vi "Check_Execution_Row.vi"(0 "Execution Row":T1 {"Row Duration (mins)" format="%#.1f"; "Row No" min=0; "Trace Gas Concentration (%)" min=0.0 format="%#.2f"; "Emission Rate (l/min)" format="%#.2f"; "Tunnel Speed" format="%#.2f"; "Start X" format="%#.2f"; "Start Y" format="%#.2f"; "Start Z" format="%#.2f"; "End X" format="%#.2f"; "End Y" format="%#.2f"; "End Z" format="%#.2f"; "Averaging time (min)" min=0.0 format="%#.2f"}, 3 "Synchronization Start No":i32=1 min=1 max=100, 4 "Row Index":i32, 5 "Max Tunnel Speed":dbl format="%.2f") -> (6 "Editted Row":bool, 7 "Execution Row Out":T1 {"Row Duration (mins)" format="%#.1f"; "Row No" min=0; "Trace Gas Concentration (%)" min=0.0 format="%#.2f"; "Emission Rate (l/min)" format="%#.2f"; "Tunnel Speed" format="%#.2f"; "Start X" format="%#.2f"; "Start Y" format="%#.2f"; "Start Z" format="%#.2f"; "End X" format="%#.2f"; "End Y" format="%#.2f"; "End Z" format="%#.2f"; "Averaging time (min)" min=0.0 format="%#.2f"}, 9 "Continue?":bool, 10 "Error Comments":string)   [LabVIEW 2012]
uses:
  Traverse_cluster.ctl
  Spacing.ctl
  Controls/Multi_run_mode.ctl
  Controls/User_Specific_mode.ctl
  Controls/Tunnel_Coordinates.ctl
  ADAM Client/Sub VIs/ADAM Controls/Channel_names.ctl
  Globals/Extra_Commands_Global.vi
  Globals/Constants_global.vi
  Globals/Trav_pos_global.vi
panel:
  out "Traverse line Out":T1 {"Row Duration (mins)" format="%#.1f"; "Row No" min=0; "Trace Gas Concentration (%)" min=0.0 format="%#.2f"; "Emission Rate (l/min)" format="%#.2f"; "Tunnel Speed" format="%#.2f"; "Start X" format="%#.2f"; "Start Y" format="%#.2f"; "Start Z" format="%#.2f"; "End X" format="%#.2f"; "End Y" format="%#.2f"; "End Z" format="%#.2f"; "Averaging time (min)" min=0.0 format="%#.2f"}
  out "Fixed Axis":bool[](array[boolean])
  out "Filenames":string[](array[string])
  out "Current Sync Number":i32
  out "Checks":string[](array[string])
  in  "Edit in Excel":bool
  in  "OK":bool
  # "X           Y            Z"
  # "Start"
  # "End"
  # "X           Y            Z"
  # "Start"
  # "End"
  # "X           Y            Z"
  # "Start"
  # "End"
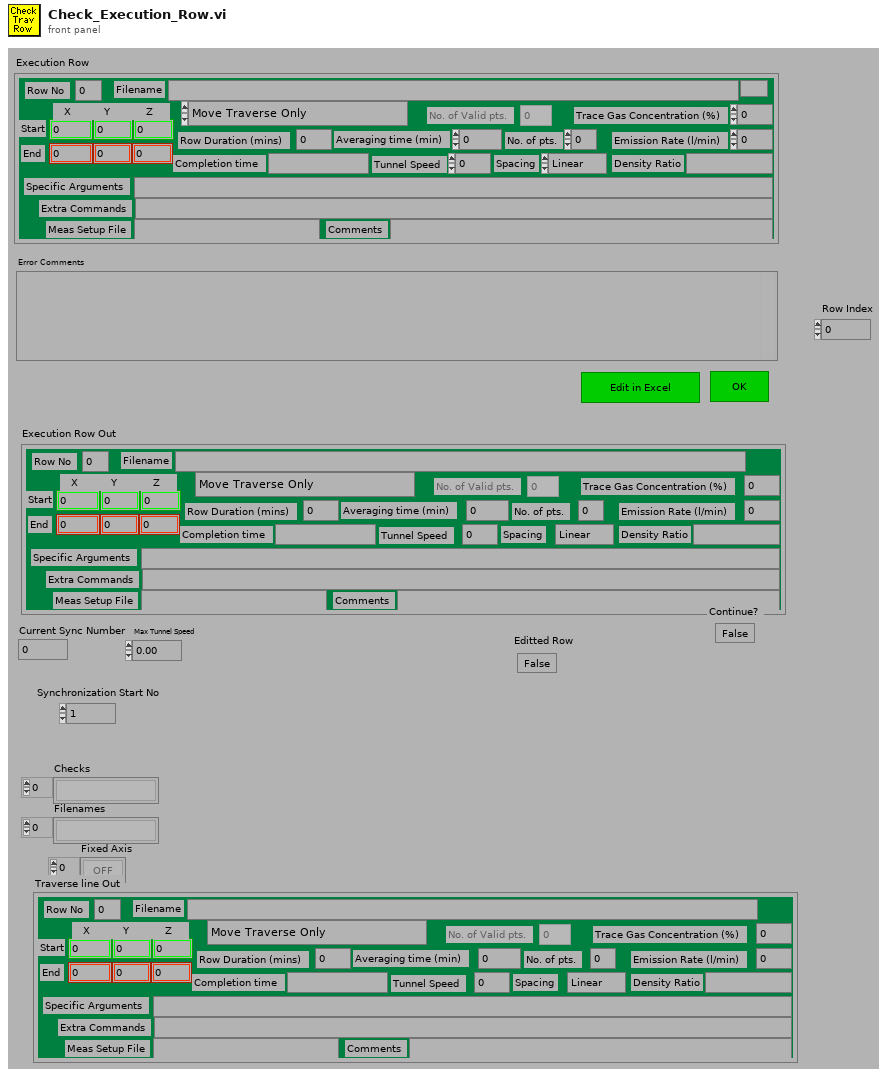
[diagram p1: front panel]
types:
  T1 = typedef "Traverse_cluster.ctl" = cluster{"Start X":dbl, "Start Y":dbl, "Start Z":dbl, "End X":dbl, "End Y":dbl, "End Z":dbl, "No. of pts.":i32, "Spacing":T2, "Filename":path, "Tunnel Speed":dbl, "Averaging time (min)":dbl, "Extra Commands":string, "Specific Arguments":string, "Emission Rate (l/min)":dbl, "Trace Gas Concentration (%)":dbl, "Density Ratio":string, "Comments":string, "Row No":i32, "Row Type Selector":T3, "Completion time":string, "Row Duration (mins)":dbl, "No. of Valid pts.":i32, "Meas Setup File":string}
  T2 = typedef "Spacing.ctl" = enum16{"Linear", "Log", "Gauss", "Specified", "N/A"}
  T3 = typedef "Multi_run_mode.ctl" = enum16{"Move Traverse Only", "Set Tunnel Speed Only", "Set Source Only", "Set Measurement Conditions", "Single Measurement", "Vertical Profile", "Lateral Profile", "Longitudinal Profile", "Explore Volume", "Multi-Axis Profile", "Auto Calibrate", "Meas Fast FID Bkgnd", "Check Beam Power", "Scanning Valve Measurement", "Run VI Named:", "Set ADAM Ch", "Wait (minutes)", "Send Message", "Synchronize With:", "Fall Back to this Row", "Turn Off Row Repeating", "Blank Row", "Traverse 3D Volume"}
  T4 = enum16{"All Channel Names", "Valid Channel Names"}
  T5 = typedef "User_Specific_mode.ctl" = enum16{"Check VI only", "Run VI"}
  T6 = typedef "Tunnel_Coordinates.ctl" = enum16{"Work in Tunnel Coordinates", "Work in Model Coordinates"}
  T7 = enum16{"Zero or one", "One", "Zero or more", "One or more"}
  T8 = typedef "Channel_names.ctl" = enum16{"Active Only", "Active + Off", "All Channels"}
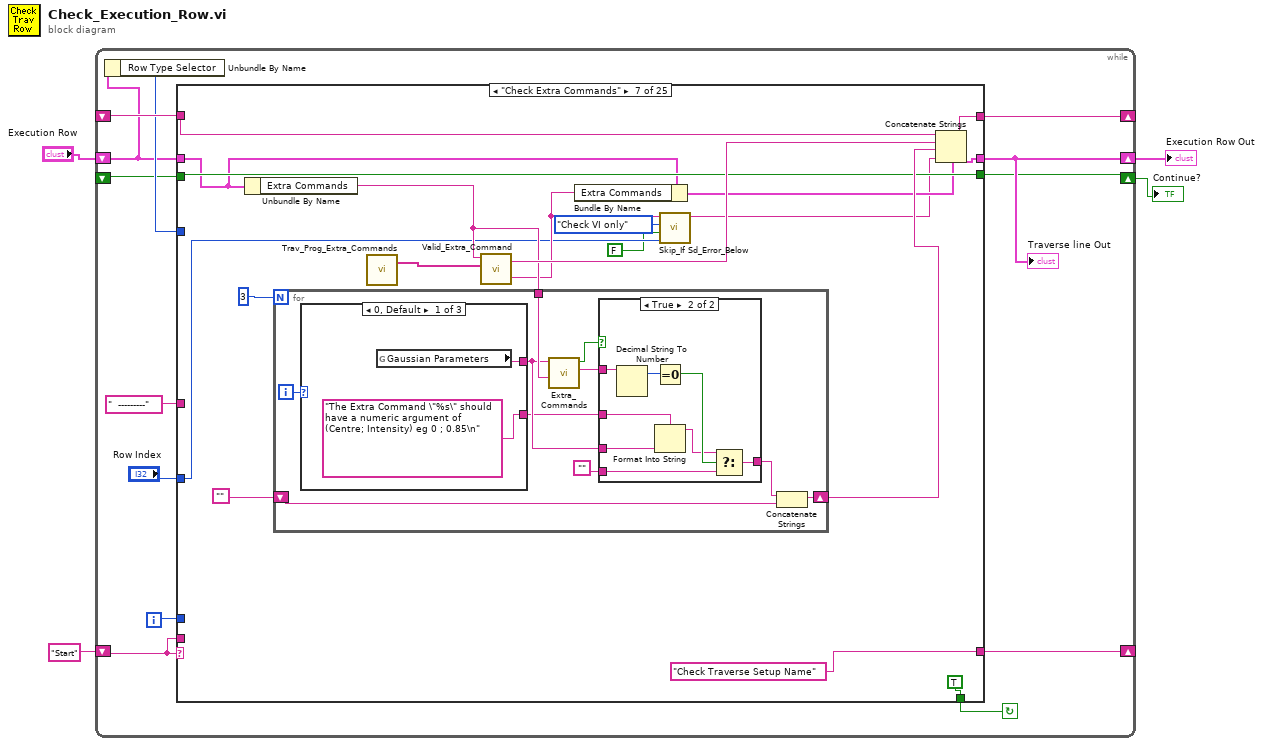
[diagram p0: block diagram]
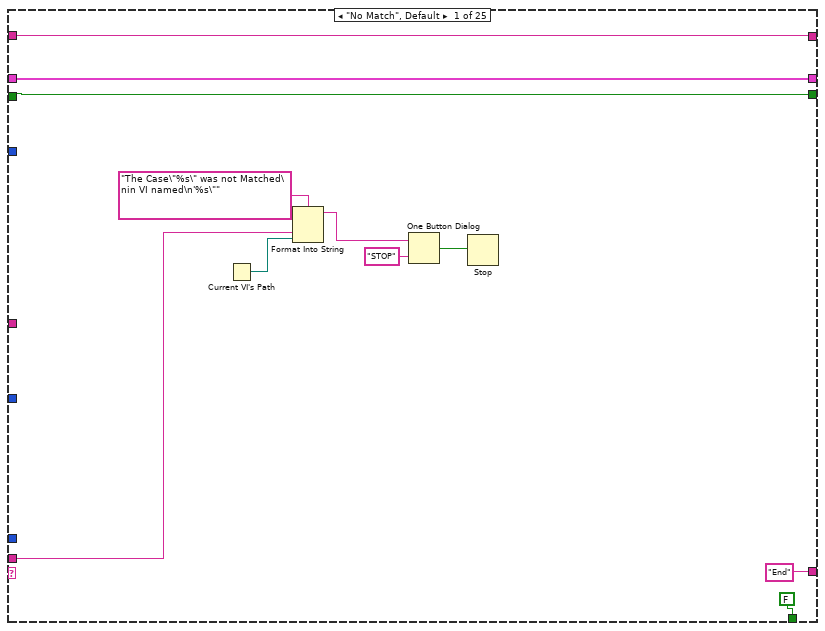
[diagram p2: hidden frame]
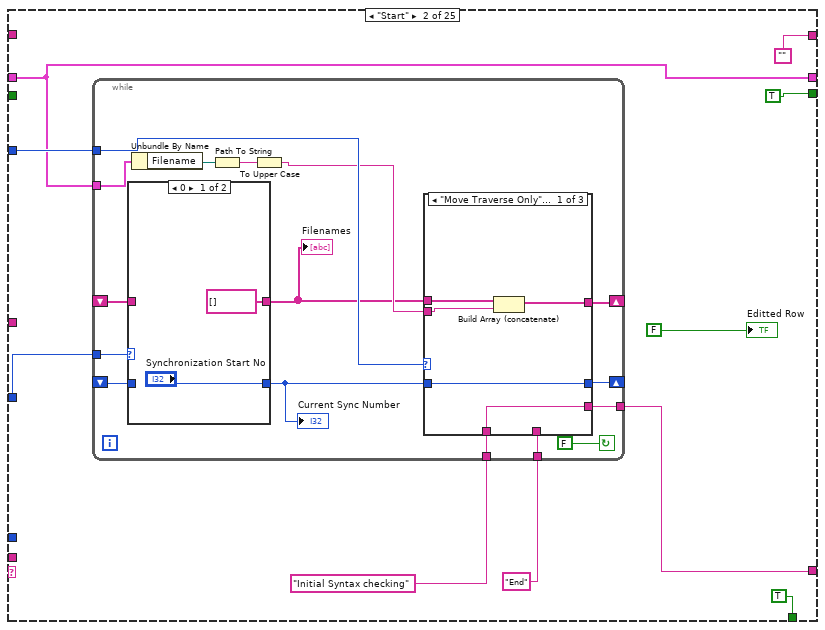
[diagram p3: hidden frame]
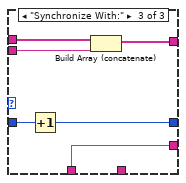
[diagram p6: hidden frame]
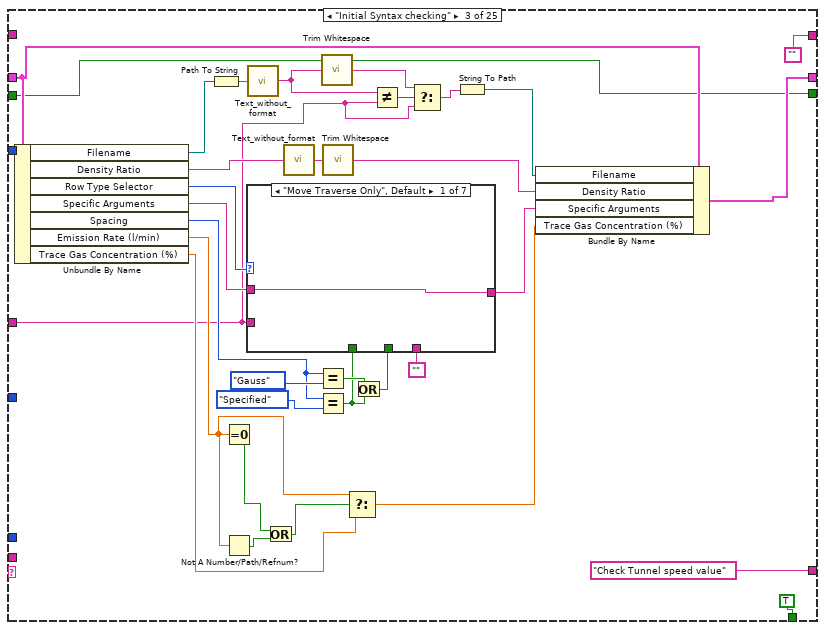
[diagram p7: hidden frame]
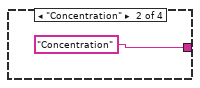
[diagram p9: hidden frame]
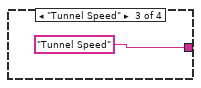
[diagram p10: hidden frame]
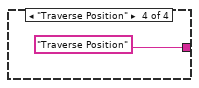
[diagram p11: hidden frame]
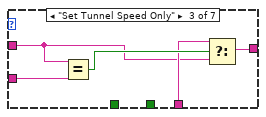
[diagram p12: hidden frame]
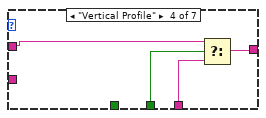
[diagram p13: hidden frame]
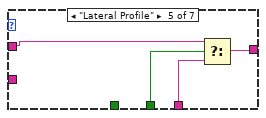
[diagram p14: hidden frame]
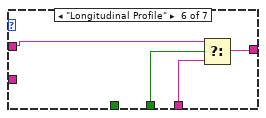
[diagram p15: hidden frame]
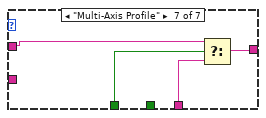
[diagram p16: hidden frame]
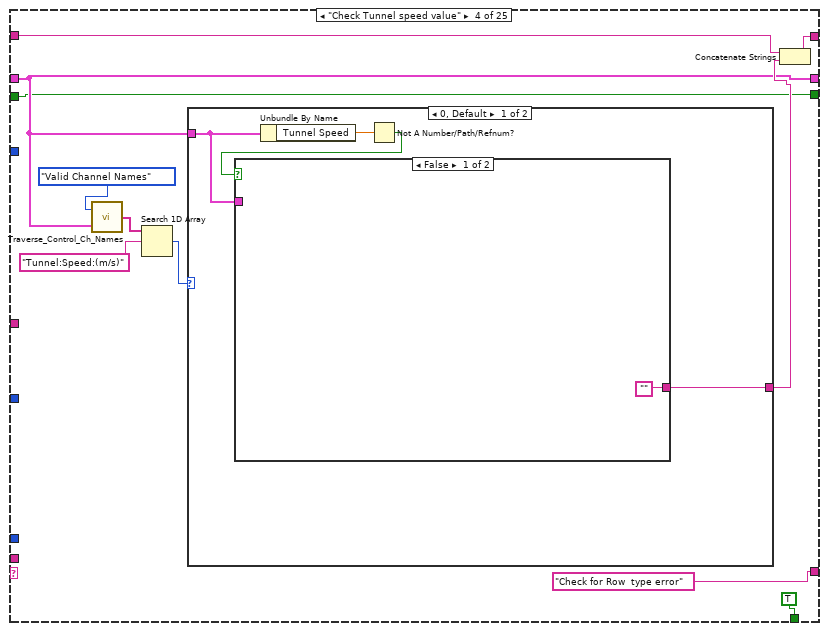
[diagram p17: hidden frame]
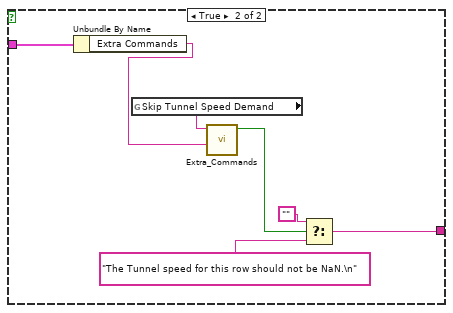
[diagram p18: hidden frame]
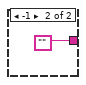
[diagram p19: hidden frame]
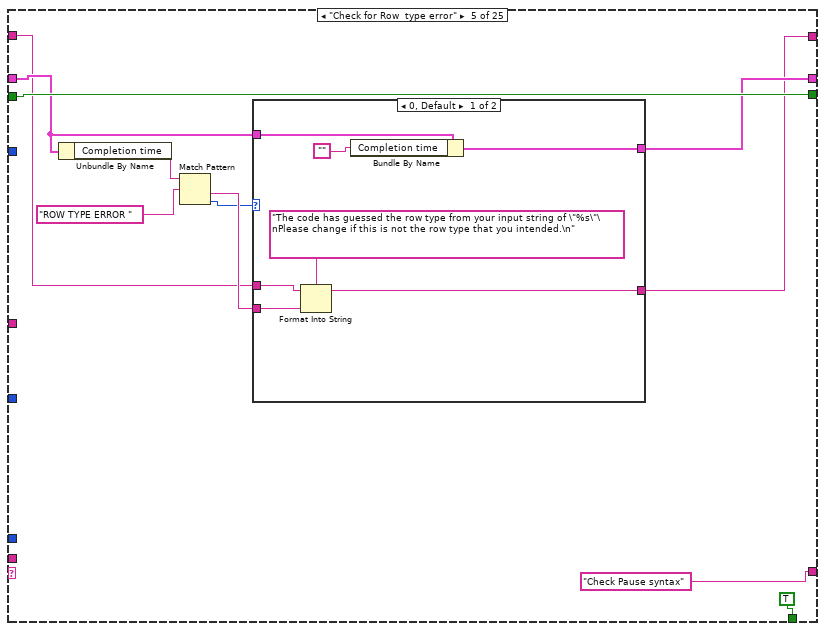
[diagram p20: hidden frame]
diagram:
  n1 = while {
    shift-left: _ -> [w16]
    shift-right: [w17] -> _
    shift-left: "Start" -> [w9]
    shift-right: [w14] -> _
    shift-right: [w8] -> w2
    shift-left: "Execution Row" -> [w5]
    shift-right: [w7] -> w1
    shift-left: _ -> [w6]
    i -> [w10]
    stop <- w15 continue-if-true
    n2 = Unbundle By Name(w5) -> ("Row Type Selector"=w12:T3)
    n3 = case shown="\"Check Extra Commands\"" w9 {
      tunnel: w5 -> [w22 w32 w100 w137 w161 w191 w205 w246 w276 w332 w365 w373 w412 w758 w858 w895 w923 w1008 w1040 w1050 w1119 _ w1158 w1165 w1175]
      tunnel: "  ---------" ("f") -> [_ _ w74 _ _ w195 _ _ _ _ _ _ _ _ _ _ _ _ _ _ _ _ _ _ _]
      tunnel: "Row Index" -> [_ w36 _ _ _ _ w202 _ _ _ _ _ w406 _ _ _ _ _ _ _ _ _ w1159 _ w1174]
      tunnel: [w21 "" "" w138 w158 w183 w213 w251 w281 w334 w369 w378 w416 w763 w868 w901 w946 w1006 w1044 w1051 w1125 w1136 w1160 w1170 w1177] -> w17
      tunnel: w12 -> [_ w35 _ _ _ _ _ _ _ _ _ w376 w415 w759 w856 _ _ _ _ w1055 _ _ _ _ _]
      tunnel: w16 -> [w21 _ _ w139 w159 w185 w214 w252 w282 w334 w368 w379 w417 w763 w869 w902 w947 w1006 w1045 w1056 w1125 w1136 w1160 w1170 w1177]
      tunnel: [FALSE TRUE TRUE TRUE TRUE TRUE TRUE TRUE TRUE TRUE TRUE TRUE TRUE TRUE TRUE TRUE TRUE TRUE TRUE w1047 TRUE TRUE TRUE TRUE FALSE] -> w15
      tunnel: ["End" w33 "Check Tunnel speed value" ("f") "Check for Row  type error" ("f") "Check Pause syntax" ("f") w188 "Check Traverse Setup Name" ("f") "Check IF command" ("f") "Check Measurement Setup?" ("f") w336 "Check Maximum tunnel speed" ("f") "Row type specific check" ("f") w413 "Check for position NaNs" ("f") w859 "Check source details" ("t") "Check source details" ("f") w1003 "check entered filename etc" ("f") w1053 "What to do next?" ("f") w1134 "Initial Syntax checking" "End" "End"] -> w14
      tunnel: w10 -> [_ _ _ _ _ _ _ _ _ _ _ _ _ _ _ _ _ _ _ _ _ _ _ _ _]
      tunnel: w9 -> [w23 _ _ _ _ _ _ _ _ _ _ _ _ _ _ _ _ _ _ _ _ _ _ _ _]
      tunnel: [w22 w32 w77 w137 w162 w178 w204 w246 w276 w332 w364 w373 w407 w757 w858 w895 w922 w1007 w1040 w1049 w1119 w1127 w1161 w1165 w1173] -> w8
      tunnel: [w18 TRUE w75 w136 w168 w179 w206 w243 w273 w338 w366 w371 w409 w755 w857 w894 w920 w1011 w1038 w1047 w1118 w1126 w1155 w1164 w1171] -> w7
      tunnel: w6 -> [w18 _ w75 w136 w168 w179 w206 w243 w273 w338 w366 w371 w409 w755 w857 w894 w920 w1011 w1038 _ w1118 _ w1155 w1164 w1171]
      frame "No Match", Default {
        n4 = Current VI's Path() -> (path=w24:path)
        n5 = Format Into String(format string="The Case\"%s\" was not Matched\nin VI named\n'%s\"" ("Format String"), w23, w24) -> (resulting string=w27:string)  [unwired: 2 in, 1 out]
        n6 = One Button Dialog(message=w27, button name ("OK")="STOP") -> (true=w25:bool)
        n7 = Stop(stop? (T)=w25) -> ()
      }
      frame "Start" {
        n8 = while {
          tunnel: "End" -> [w40]
          tunnel: "Initial Syntax checking" -> [w41]
          tunnel: [w42] -> w33
          tunnel: w32 -> [w49]
          shift-left: _ -> [w48]
          shift-right: [w47] -> _
          tunnel: w35 -> [w53]
          shift-left: _ -> [w52]
          shift-right: [w51] -> _
          tunnel: w36 -> [w54]
          stop <- FALSE continue-if-true
          n9 = case shown="0" w54 {
            tunnel: ["Synchronization Start No" w58] -> w50
            tunnel: w52 -> [_ w58]
            tunnel: w48 -> [_ w57]
            tunnel: [string[] [] w57] -> w43
            frame 0 {
            }
            frame 1, Default {
            }
          }
          "Current Sync Number" <- w50
          "Filenames" <- w43
          n10 = Unbundle By Name(w49) -> ("Filename"=w46:path)
          n11 = Path To String(path=w46) -> (string=w45:string)
          n12 = To Upper Case(1:w45) -> (0:w44:string)
          n13 = case shown="\"Move Traverse Only\", Default" w53 {
            tunnel: w50 -> [w63 w66 w72]
            tunnel: [w63 w66 w71] -> w51
            tunnel: w44 -> [w61 _ w70]
            tunnel: w43 -> [w62 w65 w69]
            tunnel: [w60 w65 w68] -> w47
            tunnel: [w59 w64 w67] -> w42
            tunnel: w41 -> [w59 _ w67]
            tunnel: w40 -> [_ w64 _]
            frame "Move Traverse Only", Default {
              n14 = Build Array (concatenate)(w62, w61) -> (w60:string[])
            }
            frame "Blank Row" {
            }
            frame "Synchronize With:" {
              n15 = Increment(x=w72) -> (x+1=w71:i32)
              n16 = Build Array (concatenate)(w69, w70) -> (w68:string[])
            }
          }
        }
        "Editted Row" <- FALSE ("Editted Row")
      }
      frame "Initial Syntax checking" {
        n17 = Unbundle By Name(w100) -> ("Filename"=w73:path, "Density Ratio"=w79:string, "Row Type Selector"=w97:T3, "Specific Arguments"=w95:string, "Spacing"=w87:T2, "Emission Rate (l/min)"=w83:dbl, "Trace Gas Concentration (%)"=w93:dbl)
        n18 = Path To String(path=w73) -> (string=w81:string)
        n19 = Equal To 0?(x=w83) -> (x = 0?=w85:bool)
        n20 = Not A Number/Path/Refnum?(number/path/refnum=w83) -> (NaN/Path/Refnum?=w84:bool)
        n21 = call "Text_without_format.vi"("Input string"=w81) -> ("Output string"=w104:string)
        n22 = Or(x=w85, y=w84) -> (x .or. y?=w82:bool)
        n23 = call "Text_without_format.vi"("Input string"=w79) -> ("Output string"=w99:string)
        n24 = Equal?(x=w87, y=Spacing."Gauss" ("Spacing")) -> (x = y?=w89:bool)
        n25 = Equal?(x=w87, y=Spacing."Specified" ("Spacing")) -> (x = y?=w86:bool)
        n26 = call <vilib>:"Trim Whitespace.vi"("string"=w104) -> ("trimmed string"=w103:string)  [unwired: 1 in]
        n27 = call <vilib>:"Trim Whitespace.vi"("string"=w99) -> ("trimmed string"=w78:string)  [unwired: 1 in]
        n28 = Select(t=w83, s=w82, f=w93) -> (s? t:f=w92:dbl)
        n29 = Or(x=w89, y=w86) -> (x .or. y?=w88:bool)
        n30 = case shown="\"Move Traverse Only\", Default" w97 {
          tunnel: [w106 w108 w113 w119 w123 w127 w131] -> w96
          tunnel: w95 -> [w106 w107 w114 w121 w125 w129 w133]
          tunnel: "" -> [_ _ w115 w120 w124 w128 w132]
          tunnel: w88 -> [_ _ _ w118 w122 w126 _]
          tunnel: w86 -> [_ _ _ _ _ _ w130]
          tunnel: w74 -> [_ _ w117 _ _ _ _]
          frame "Move Traverse Only", Default {
          }
          frame "Auto Calibrate" {
            n31 = case shown="\"No Match\", Default" w107 {
              tunnel: [w109 "Concentration" "Tunnel Speed" "Traverse Position"] -> w108
              tunnel: w107 -> [w109 _ _ _]
              frame "No Match", Default {
              }
              frame "Concentration" {
              }
              frame "Tunnel Speed" {
              }
              frame "Traverse Position" {
              }
            }
          }
          frame "Set Tunnel Speed Only" {
            n32 = Equal?(x=w114, y=w117) -> (x = y?=w116:bool)
            n33 = Select(t=w115, s=w116, f=w114) -> (s? t:f=w113:string)
          }
          frame "Vertical Profile" {
            n34 = Select(t=w121, s=w118, f=w120) -> (s? t:f=w119:string)
          }
          frame "Lateral Profile" {
            n35 = Select(t=w125, s=w122, f=w124) -> (s? t:f=w123:string)
          }
          frame "Longitudinal Profile" {
            n36 = Select(t=w129, s=w126, f=w128) -> (s? t:f=w127:string)
          }
          frame "Multi-Axis Profile" {
            n37 = Select(t=w133, s=w130, f=w132) -> (s? t:f=w131:string)
          }
        }
        n38 = Not Equal?(x=w104, y=w74) -> (x != y?=w105:bool)
        n39 = Select(t=w103, s=w105, f=w74) -> (s? t:f=w102:string)
        n40 = String To Path(string=w102) -> (path=w80:path)
        n41 = Bundle By Name(cluster=w100, "Filename"=w80, "Density Ratio"=w78, "Specific Arguments"=w96, "Trace Gas Concentration (%)"=w92) -> (w77:T1)
      }
      frame "Check Tunnel speed value" {
        n42 = call "Traverse_Control_Ch_Names.vi"("Traverse line"=w137, "Mode"=T4."Valid Channel Names") -> ("Channel names"=w143:string[])
        n43 = Search 1D Array(1D array=w143, element="Tunnel:Speed:(m/s)" ("Label for value")) -> (index of element=w141:i32)  [unwired: 1 out]
        n44 = case shown="0, Default" w141 {
          tunnel: w137 -> [w146 _]
          tunnel: [w145 ""] -> w140
          frame 0, Default {
            n45 = Unbundle By Name(w146) -> ("Tunnel Speed"=w148:dbl)
            n46 = Not A Number/Path/Refnum?(number/path/refnum=w148) -> (NaN/Path/Refnum?=w147:bool)
            n47 = case shown="False" w147 {
              tunnel: w146 -> [_ w156]
              tunnel: ["" w150] -> w145
              frame False {
              }
              frame True {
                n48 = Unbundle By Name(w156) -> ("Extra Commands"=w154:string)
                n49 = global read "Extra_Commands_Global.vi" "Skip Tunnel Speed Demand"() -> (w155:string)
                n50 = call "Extra_Commands.vi"("String to Search"=w154, "Command"=w155) -> ("Command Found"=w153:bool)  [unwired: 1 in, 4 out]
                n51 = Select(t="", s=w153, f="The Tunnel speed for this row should not be NaN.\n") -> (s? t:f=w150:string)
              }
            }
          }
          frame -1 {
          }
        }
        n52 = Concatenate Strings(w139, w140) -> (w138:string)
      }
      frame "Check for Row  type error" {
        n53 = Unbundle By Name(w161) -> ("Completion time"=w164:string)
        n54 = Match Pattern(string=w164, regular expression="ROW TYPE ERROR " ("format string")) -> (after substring=w163:string, offset past match=w160:i32)  [unwired: 3 out]
        n55 = case shown="0, Default" w160 {
          tunnel: w163 -> [w175 _]
          tunnel: [w173 w177] -> w162
          tunnel: w161 -> [w172 w177]
          tunnel: [w170 w176] -> w158
          tunnel: w159 -> [w169 w176]
          frame 0, Default {
            n56 = Format Into String(format string="The code has guessed the row type from your input string of \"%s\"\nPlease change if this is not the row type that you intended.\n", initial string=w169, w175) -> (resulting string=w170:string)  [unwired: 1 in, 1 out]
            n57 = Bundle By Name(cluster=w172, "Completion time"="") -> (w173:T1)
          }
          frame -1 {
          }
        }
      }
      frame "Check Pause syntax" {
        n58 = Unbundle By Name(w191) -> ("Extra Commands"=w196:string)
        n59 = Not Equal?(x=w196, y=w195) -> (x != y?=w197:bool)
        n60 = Select(t=w196, s=w197, f="") -> (s? t:f=w193:string)
        n61 = call <vilib>:"Trim Whitespace.vi"("string"=w193) -> ("trimmed string"=w187:string)  [unwired: 1 in]
        n62 = Equal?(x=w187, y="") -> (x = y?=w189:bool)
        n63 = call "Pause_for_server_ch_val.vi"("Extra command string"=w187, "Simulate/Run"=User_Specific_mode."Check VI only") -> ("Extra command string Out"=w186:string, "Error Comments"=w184:string)
        n64 = Bundle By Name(cluster=w191, "Extra Commands"=w186) -> (w178:T1)
        n65 = Concatenate Strings(w185, w184) -> (w183:string)
        n66 = Select(t="Check Measurement Setup?", s=w189, f="Check Extra Commands") -> (s? t:f=w188:string)
      }
      frame "Check Extra Commands" {
        n67 = Unbundle By Name(w205) -> ("Extra Commands"=w207:string)
        n68 = for {
          N: 3 -> [_]
          tunnel: w207 -> [w222]
          shift-right: [w218] -> w210
          shift-left: "" -> [w219]
          i -> [w224]
          n69 = case shown="0, Default" w224 {
            tunnel: [w227 w229 w231] -> w221
            tunnel: ["The Extra Command \"%s\" should have a numeric argument of (Centre; Intensity) eg 0 ; 0.85\n" ("Format String") "The Extra Command \"%s\" should have a numeric argument.\n" ("Format String") "The Extra Command \"%s\" should have a numeric argument.\n" ("Format String")] -> w216
            frame 0, Default {
              n70 = global read "Extra_Commands_Global.vi" "Gaussian Parameters"() -> (w227:string)
            }
            frame 1 {
              n71 = global read "Extra_Commands_Global.vi" "Establish Exp Conditions (s)"() -> (w229:string)
            }
            frame 2 {
              n72 = global read "Extra_Commands_Global.vi" "Minutes Before Repeating Row"() -> (w231:string)
            }
          }
          n73 = call "Extra_Commands.vi"("String to Search"=w222, "Command"=w221) -> ("String Value"=w223:string, "Command Found"=w225:bool)  [unwired: 1 in, 3 out]
          n74 = case shown="True" w225 {
            tunnel: w223 -> [_ w240]
            tunnel: w221 -> [_ w238]
            tunnel: [w232 w235] -> w220
            tunnel: "" -> [w232 w234]
            tunnel: w216 -> [_ w233]
            frame False {
            }
            frame True {
              n75 = Decimal String To Number(string=w240) -> (offset past number=w239:i32)  [unwired: 3 out]
              n76 = Equal To 0?(x=w239) -> (x = 0?=w237:bool)
              n77 = Format Into String(format string=w233, w238) -> (resulting string=w236:string)  [unwired: 2 in, 1 out]
              n78 = Select(t=w236, s=w237, f=w234) -> (s? t:f=w235:string)
            }
          }
          n79 = Concatenate Strings(w220, w219) -> (w218:string)
        }
        n80 = call "Trav_Prog_Extra_Commands.vi"() -> ("Extra Commands Array"=w208:string[])  [unwired: 2 out]
        n81 = call "Valid_Extra_Command.vi"("Extra Commands string"=w207, "Valid Commands Array"=w208) -> ("Output String"=w212:string, "Extra Commands string Out"=w203:string)  [unwired: 3 out]
        n82 = Bundle By Name(cluster=w205, "Extra Commands"=w203) -> (w204:T1)
        n83 = call "Skip_If Sd_Error_Below.vi"("String to Search"=w203, "Simulate/Run"=User_Specific_mode."Check VI only", "Measurement setup Applied?"=FALSE, "Row Number"=w202) -> ("Error String"=w199:string)  [unwired: 1 in, 4 out]
        n84 = Concatenate Strings(w214, w212, w210, w199) -> (w213:string)
      }
      frame "Check Traverse Setup Name" {
        n85 = Unbundle By Name(w246) -> ("Extra Commands"=w242:string)
        n86 = global read "Extra_Commands_Global.vi" "!Traverse Setup"() -> (w249:string)
        n87 = call "Extra_Commands.vi"("String to Search"=w242, "Command"=w249) -> ("String Value"=w247:string, "Command Found"=w248:bool)  [unwired: 1 in, 3 out]
        n88 = case shown="True" w248 {
          tunnel: w247 -> [_ w259]
          tunnel: [w253 w256] -> w244
          tunnel: "" -> [w253 w255]
          frame False {
          }
          frame True {
            n89 = global read "Constants_global.vi" "Traverse folder"() -> (w254:path)
            n90 = List Folder(path=w254) -> (folder names=w257:string[])  [unwired: 1 in, 5 out]
            n91 = Search 1D Array(1D array=w257, element=w259) -> (index of element=w260:i32)  [unwired: 1 out]
            n92 = Greater Or Equal To 0?(x=w260) -> (x >= 0?=w258:bool)
            n93 = case shown="False" w258 {
              tunnel: w259 -> [w265 _]
              tunnel: w257 -> [w262 _]
              tunnel: [w261 w270] -> w256
              tunnel: w255 -> [_ w270]
              frame False {
                n94 = Format Into String(format string="%s is not a valid Travese setup. Valid option are:", w265) -> (resulting string=w263:string)  [unwired: 2 in, 1 out]
                n95 = for {
                  shift-right: [w267] -> w261
                  shift-left: w263 -> [w268]
                  tunnel: w262 -> [w269] mode=indexing
                  w266 = "  " ("Substring")
                  n96 = Concatenate Strings(w268, w266, w269, w266) -> (w267:string)
                }
              }
              frame True {
              }
            }
          }
        }
        n97 = Concatenate Strings(w252, w244) -> (w251:string)
      }
      frame "Check IF command" {
        n98 = Unbundle By Name(w276) -> ("Extra Commands"=w272:string)
        n99 = global read "Extra_Commands_Global.vi" "If Command"() -> (w279:string)
        n100 = call "Extra_Commands.vi"("String to Search"=w272, "Command"=w279) -> ("String Value"=w277:string, "Command Found"=w278:bool)  [unwired: 1 in, 3 out]
        n101 = case shown="True" w278 {
          tunnel: w277 -> [_ w288]
          tunnel: [w283 w287] -> w274
          tunnel: "" -> [w283 w285]
          frame False {
          }
          frame True {
            n102 = call "Get_array_values_fr_String.vi"("String Value"=w288) -> ("Numeric Array"=w284:dbl[], "String array"=w286:string[])
            n103 = Index Array(array=w286, index=0 ("Index")) -> (element=w289:string)
            n104 = case shown="\"Global Value Between\"" w289 {
              tunnel: w288 -> [w294 _ _ _]
              tunnel: [w293 w319 w320 "The !If  command has not been recognised.\nExtra command Example:\n!IF = Time Between;10:45;and;14:00;Execute Row (or) Skip Row\n\n!IF = ADAM Channel Between;Channel Name; 0.5;1.0\n\n!IF = Global Value Between; 0.5;1.0" ("Error Comments")] -> w287
              tunnel: w286 -> [_ w310 w328 _]
              tunnel: w285 -> [_ w303 w321 _]
              tunnel: w284 -> [_ _ _ _]
              frame "Time Between" {
                n105 = Get Date/Time In Seconds() -> (seconds since 1Jan1904=w291:timestamp)
                n106 = To Double Precision Float(number=w291) -> (double precision float=w292:dbl)
                n107 = call "If_Time_arguments.vi"("seconds since 1Jan1904"=w292, "String Value"=w294) -> ("Error Comments"=w293:string)  [unwired: 2 out]
              }
              frame "ADAM Channel Between" {
                n108 = Index Array(array=w310, index=1 ("Index")) -> (element=w313:string)
                n109 = Index Array(array=w310, index=2 ("Index")) -> (element=w309:string)
                n110 = Index Array(array=w310, index=3 ("Index")) -> (element=w308:string)
                n111 = Build Array(w313) -> (w315:string[])
                n112 = Decimal Digit?(1:w309) -> (0:w306:bool)
                n113 = Decimal Digit?(1:w308) -> (0:w307:bool)
                n114 = call "Get_Current_Scan_client.vi"("ADAM Ch Names"=w315) -> ("Numerical Values"=w317:dbl[])  [unwired: 3 out]
                n115 = And(x=w306, y=w307) -> (x .and. y?=w305:bool)
                n116 = Index Array(array=w317, index=0 ("Index")) -> (element=w318:dbl)
                n117 = Select(t=w303, s=w305, f="you must give two limits\n") -> (s? t:f=w299:string)
                n118 = Not A Number/Path/Refnum?(number/path/refnum=w318) -> (NaN/Path/Refnum?=w302:bool)
                n119 = Select(t="Invalid ADAM Channel Name\n", s=w302, f=w303) -> (s? t:f=w300:string)
                n120 = Concatenate Strings(w300, w299) -> (w297:string)
                n121 = Concatenate Strings(w297, "Extra command Example:\n!IF = ADAM Channel Between;Channel Name; 0.5;1.0") -> (w296:string)
                n122 = Empty String/Path?(string/path=w297) -> (empty?=w298:bool)
                n123 = Select(t=w303, s=w298, f=w296) -> (s? t:f=w319:string)
              }
              frame "Global Value Between" {
                n124 = Index Array(array=w328, index=1 ("Index")) -> (element=w327:string)
                n125 = Index Array(array=w328, index=2 ("Index")) -> (element=w326:string)
                n126 = Decimal Digit?(1:w327) -> (0:w324:bool)
                n127 = Decimal Digit?(1:w326) -> (0:w325:bool)
                n128 = And(x=w324, y=w325) -> (x .and. y?=w323:bool)
                n129 = Select(t=w321, s=w323, f="The Extra command IF statement must have two numerical values for the limits\n\nExtra command Example:\n!IF = Global Value Between; 0.5;1.0") -> (s? t:f=w320:string)
              }
              frame "No Match", Default {
              }
            }
          }
        }
        n130 = Concatenate Strings(w282, w274) -> (w281:string)
      }
      frame "Check Measurement Setup?" {
        n131 = Unbundle By Name(w332) -> ("Row Type Selector"=w337:T3, "Specific Arguments"=w335:string)
        n132 = case shown="\"Traverse 3D Volume\"" w337 {
          tunnel: ["Check Measurement Setup" ("t") "Check Measurement Setup" ("t") "Check Measurement Setup" ("t") "Check Measurement Setup" ("t") "Check Measurement Setup" ("t") "Check Measurement Setup" ("t") "Check Measurement Setup" ("t") "Check Measurement Setup" ("t") "Check Measurement Setup" ("t") "Check Measurement Setup" ("t") "Check Measurement Setup" ("t") w351 w360] -> w336
          tunnel: w335 -> [_ _ _ _ _ _ _ _ _ _ _ w358 _]
          tunnel: "Check Maximum tunnel speed" ("f") -> [_ _ _ _ _ _ _ _ _ _ _ w352 w360]
          tunnel: w332 -> [_ _ _ _ _ _ _ _ _ _ _ w355 _]
          frame "Lateral Profile" {
          }
          frame "Traverse 3D Volume" {
          }
          frame "Longitudinal Profile" {
          }
          frame "Explore Volume" {
          }
          frame "Multi-Axis Profile" {
          }
          frame "Vertical Profile" {
          }
          frame "Single Measurement" {
          }
          frame "Scanning Valve Measurement" {
          }
          frame "Auto Calibrate" {
          }
          frame "Meas Fast FID Bkgnd" {
          }
          frame "Check Beam Power" {
          }
          frame "Run VI Named:" {
            n133 = Match Pattern(string=w358, regular expression=";") -> (before substring=w357:string)  [unwired: 4 out]
            n134 = call <vilib>:"Trim Whitespace.vi"("string"=w357) -> ("trimmed string"=w356:string)  [unwired: 1 in]
            n135 = call "Run_VI_Named_specific.vi"("Run VI Named String"=w356, "Multi Run Row"=w355) -> ("Check Meas Setup?"=w354:bool)  [unwired: 9 out]
            n136 = Select(t="Check Measurement Setup", s=w354, f=w352) -> (s? t:f=w351:string)
          }
          frame "Set Tunnel Speed Only", Default {
          }
        }
      }
      frame "Check Measurement Setup" {
        n137 = Unbundle By Name(w365) -> ("Meas Setup File"=w363:string)
        n138 = call "Check_Measurement_Setups.vi"("Measurement Setup String"=w363) -> ("Measurement Setup String Out"=w362:string, "Error Comments"=w361:string)
        n139 = Bundle By Name(cluster=w365, "Meas Setup File"=w362) -> (w364:T1)
        n140 = Concatenate Strings(w368, w361) -> (w369:string)
      }
      frame "Check Maximum tunnel speed" {
        n141 = case shown="\"Set Tunnel Speed Only\", Default" w376 {
          tunnel: w373 -> [w398 _]
          tunnel: [w389 FALSE] -> w375
          tunnel: [w388 0.0] -> w374
          frame "Auto Calibrate" {
            n142 = Unbundle By Name(w398) -> ("Specific Arguments"=w397:string)
            n143 = call "Get_array_values_fr_String.vi"("String Value"=w397) -> ("Numeric Array"=w391:dbl[], "String array"=w396:string[])
            n144 = Index Array(array=w396, index=0 ("Index")) -> (element=w394:string)
            n145 = Equal?(x=w394, y="Tunnel Speed" ("Output Array")) -> (x = y?=w389:bool)
            n146 = Array Subset(array=w391, index=1 ("Array Index")) -> (w390:dbl[])  [unwired: 1 in]
            n147 = Array Max & Min(array=w390) -> (max value=w388:dbl)  [unwired: 3 out]
          }
          frame "Set Tunnel Speed Only", Default {
          }
        }
        n148 = case shown="False" w375 {
          tunnel: [w386 w387] -> w383
          tunnel: w373 -> [w385 _]
          tunnel: w374 -> [_ w387]
          frame False {
            n149 = Unbundle By Name(w385) -> ("Tunnel Speed"=w386:dbl)
          }
          frame True {
          }
        }
        n150 = Greater?(x=w383, y="Max Tunnel Speed") -> (0:w381:bool)
        n151 = Not A Number/Path/Refnum?(number/path/refnum=w383) -> (NaN/Path/Refnum?=w382:bool)
        n152 = Compound Arithmetic op=AND(invert w382, w381) -> (w380:bool)
        n153 = case shown="False" w380 {
          tunnel: w379 -> [w401 w403]
          tunnel: [w401 w402] -> w378
          tunnel: "Max Tunnel Speed" -> [_ w405]
          frame False {
          }
          frame True {
            n154 = Format Into String(format string="The maximum allowable tunnel speed is %.2f m/s.\n" ("Format String"), initial string=w403, w405) -> (resulting string=w402:string)  [unwired: 1 in, 1 out]
          }
        }
      }
      frame "Row type specific check" {
        n155 = case shown="\"Check Beam Power\"" w415 {
          tunnel: w412 -> [w426 w435 w439 w443 w448 w453 w460 w467 w478 w486 w500 w504 w581 w588 w609 w637 w686 w714 w719 w723 w735 w739 w745]
          tunnel: [string[] [] string[] [] string[] [] string[] [] w449 w456 w463 w470 w483 w491 w501 w526 w583 string[] [] w626 string[] [] w681 string[] [] string[] [] string[] [] string[] [] string[] [] string[] []] -> w414
          tunnel: [w420 "" "" "" "" "" "" "" w479 w488 "" w540 w577 w587 w621 w629 w697 w716 "" w725 "" "" w747] -> w418
          tunnel: [w429 w436 w440 w444 w447 w454 w461 w468 w477 w487 w499 w525 w571 w586 w620 w640 w682 "check entered filename etc" "check entered filename etc" "check entered filename etc" "check entered filename etc" "check entered filename etc" "check entered filename etc"] -> w413
          tunnel: "Check source details" -> [_ w436 w440 _ _ _ _ _ _ _ w499 _ w571 w586 w620 w639 w683 _ _ _ _ _ _]
          tunnel: "Sort out start and end positions" -> [_ _ _ _ _ w454 w461 w468 _ w487 _ w523 _ _ _ _ _ _ _ _ _ _ _]
          tunnel: "Check for Start NaNs" -> [w429 _ _ w444 w447 _ _ _ w477 _ _ w524 _ _ _ _ _ _ _ _ _ _ _]
          tunnel: [w425 w435 w439 w443 w448 w453 w460 w467 w478 w486 w500 w505 w581 w596 w609 w636 w686 w714 w719 w723 w735 w739 w743] -> w407
          tunnel: w406 -> [_ _ _ _ _ _ _ _ _ _ _ _ _ _ _ w642 _ _ _ _ _ _ _]
          frame "Move Traverse Only" {
            n156 = Unbundle By Name(w426) -> ("Specific Arguments"=w427:string)
            n157 = call <vilib>:"Trim Whitespace.vi"("string"=w427) -> ("trimmed string"=w421:string)  [unwired: 1 in]
            n158 = Equal?(x=w421, y="No Backlash") -> (x = y?=w424:bool)
            n159 = Empty String/Path?(string/path=w421) -> (empty?=w423:bool)
            n160 = Or(x=w423, y=w424) -> (x .or. y?=w422:bool)
            n161 = case shown="True" w422 {
              tunnel: w421 -> [w432 _]
              tunnel: [w431 ""] -> w420
              frame False {
                n162 = Format Into String(format string="\"%s\" is an Incorrect Specific Argument. It should either be left blank or say \"No Backlash\"\n", w432) -> (resulting string=w431:string)  [unwired: 2 in, 1 out]
              }
              frame True {
              }
            }
            n163 = Bundle By Name(cluster=w426, "Specific Arguments"=w421) -> (w425:T1)
          }
          frame "Set Tunnel Speed Only" {
          }
          frame "Set Source Only" {
          }
          frame "Set Measurement Conditions" {
          }
          frame "Single Measurement" {
            n164 = Build Array("Averaging:Time:(mins)" ("Label for value"), "Filename:HD:Users" ("Label for value")) -> (w449:string[])
          }
          frame "Vertical Profile" {
            n165 = Build Array("Number:Of:Points" ("Label for value"), "Averaging:Time:(mins)" ("Label for value"), "Filename:HD:Users" ("Label for value")) -> (w456:string[])
          }
          frame "Lateral Profile" {
            n166 = Build Array("Number:Of:Points" ("Label for value"), "Averaging:Time:(mins)" ("Label for value"), "Filename:HD:Users" ("Label for value")) -> (w463:string[])
          }
          frame "Longitudinal Profile" {
            n167 = Build Array("Number:Of:Points" ("Label for value"), "Averaging:Time:(mins)" ("Label for value"), "Filename:HD:Users" ("Label for value")) -> (w470:string[])
          }
          frame "Explore Volume" {
            n168 = Unbundle By Name(w478) -> ("Specific Arguments"=w476:string)
            n169 = Build Array("Averaging:Time:(mins)" ("Label for value"), "Filename:HD:Users" ("Label for value")) -> (w483:string[])
            n170 = Fract/Exp String To Number(string=w476) -> (number=w475:dbl)  [unwired: 4 out]
            n171 = Greater Than 0?(x=w475) -> (x > 0?=w474:bool)
            n172 = Format Into String(format string="\"%s\" is an Incorrect Specific Argument. Please enter the radius of the volume in mm.\n", w476) -> (resulting string=w480:string)  [unwired: 2 in, 1 out]
            n173 = Select(t="", s=w474, f=w480) -> (s? t:f=w479:string)
          }
          frame "Multi-Axis Profile" {
            n174 = Unbundle By Name(w486) -> ("Spacing"=w489:T2)
            n175 = case shown="\"Gauss\"" w489 {
              tunnel: ["" "You are not allowed to specify gaussian spacing for a Multi-Axis profile.\n" "You are not allowed to specify Log spacing for a Multi-Axis profile.\n" "\"N/A\" is not a valid point spacing.\n"] -> w488
              frame "Linear", Default {
              }
              frame "Gauss" {
              }
              frame "Log" {
              }
              frame "N/A" {
              }
            }
            n176 = Build Array("Number:Of:Points" ("Label for value"), "Averaging:Time:(mins)" ("Label for value"), "Filename:HD:Users" ("Label for value")) -> (w491:string[])
          }
          frame "Traverse 3D Volume" {
            n177 = Build Array("Averaging:Time:(mins)" ("Label for value"), "Filename:HD:Users" ("Label for value")) -> (w501:string[])
          }
          frame "Auto Calibrate" {
            n178 = Unbundle By Name(w504) -> ("Filename"=w508:path, "Specific Arguments"=w539:string)
            n179 = call "Get_array_values_fr_String.vi"("String Value"=w539) -> ("Numeric Array"=w535:dbl[], "String array"=w522:string[])
            n180 = global read "Trav_pos_global.vi" "Work in Tunnel Coordinates?"() -> (w518:T6)
            n181 = Index Array(array=w522, index=0 ("Index")) -> (element=w521:string)
            n182 = Build Array("Tunnel Speed", "Traverse Position", "Concentration") -> (w520:string[])
            n183 = Build Array("Averaging:Time:(mins)" ("Label for value")) -> (w526:string[])
            n184 = Array Size(array=w535) -> (size(s)=w534:i32)
            n185 = call "Current_Filepath.vi"("Filename in"=w508, "Data Type"="Calibrations") -> ("Filename Out"=w506:path)  [unwired: 1 out]
            n186 = Equal?(x=w518, y=Tunnel_Coordinates."Work in Model Coordinates" ("Work in Tunnel Coordinates?")) -> (x = y?=w512:bool)
            n187 = Search 1D Array(1D array=w520, element=w521) -> (index of element=w513:i32)  [unwired: 1 out]
            n188 = Equal?(x=2, y=w513) -> (x = y?=w515:bool)
            n189 = case shown="1" w513 {
              tunnel: [w569 w570] -> w525
              tunnel: w524 -> [w569 _]
              tunnel: w523 -> [_ w570]
              frame 0, Default {
              }
              frame 1 {
              }
            }
            n190 = Less?(x=w534, y=3) -> (x < y?=w530:bool)
            n191 = Equal To 0?(x=w513) -> (x = 0?=w531:bool)
            n192 = And(x=w512, y=w515) -> (x .and. y?=w514:bool)
            n193 = Greater Or Equal To 0?(x=w513) -> (x >= 0?=w511:bool)
            n194 = Compound Arithmetic op=AND(w530, w531) -> (w529:bool)
            n195 = case shown="True" w514 {
              tunnel: [w556 w561] -> w507
              tunnel: w504 -> [w556 w557]
              frame False {
              }
              frame True {
                n196 = global read "Extra_Commands_Global.vi" "Work in Tunnel Coordinates"() -> (w559:string)
                n197 = Unbundle By Name(w557) -> ("Extra Commands"=w558:string)
                n198 = call "Extra_Commands.vi"("String to Search"=w558, "Command"=w559) -> ("Command Found"=w560:bool)  [unwired: 1 in, 4 out]
                n199 = case shown="False" w560 {
                  tunnel: [w567 w568] -> w561
                  tunnel: w559 -> [w566 _]
                  tunnel: w558 -> [w565 _]
                  tunnel: w557 -> [w563 w568]
                  frame False {
                    n200 = Concatenate Strings(w566, "  " ("string"), w565) -> (w564:string)
                    n201 = Bundle By Name(cluster=w563, "Extra Commands"=w564) -> (w567:T1)
                  }
                  frame True {
                  }
                }
              }
            }
            n202 = Select(t="You need to enter the desired tunnel speeds in the \"Specfic Arguments\" Box   eg.  Tunnel Speed;1;2;3;4\n", s=w529, f="") -> (s? t:f=w527:string)
            n203 = call "Does_file_exist_(simple).vi"("Pathname"=w506) -> ("exists?"=w545:bool)
            n204 = case shown="False" w511 {
              tunnel: w520 -> [w547 _]
              tunnel: [w546 ""] -> w510
              frame False {
                n205 = for {
                  shift-right: [w552] -> w549
                  shift-left: "Incorrect Specific Argument. The options are: " -> [w553]
                  tunnel: w547 -> [w554] mode=indexing
                  w551 = "  " ("Substring")
                  n206 = Concatenate Strings(w553, w551, w554, w551) -> (w552:string)
                }
                n207 = Concatenate Strings(w549, "\r\n") -> (w546:string)
              }
              frame True {
              }
            }
            n208 = Select(t="", s=w545, f="The calibration file cannot be found.\n") -> (s? t:f=w541:string)
            n209 = Bundle By Name(cluster=w507, "Filename"=w506) -> (w505:T1)
            n210 = Concatenate Strings(w541, w527, w510) -> (w540:string)
          }
          frame "Meas Fast FID Bkgnd" {
            n211 = Unbundle By Name(w581) -> ("Specific Arguments"=w576:string)
            n212 = call "Get_array_values_fr_String.vi"("String Value"=w576) -> ("String array"=w575:string[])  [unwired: 1 out]
            n213 = Index Array(array=w575, index=0) -> (element=w573:string)
            n214 = Empty String/Path?(string/path=w573) -> (empty?=w579:bool)
            n215 = Build Array("Averaging:Time:(mins)" ("Label for value")) -> (w583:string[])
            n216 = Equal?(x=w573, y="Use Source Divertor Valve") -> (x = y?=w572:bool)
            n217 = Or(x=w579, y=w572) -> (x .or. y?=w578:bool)
            n218 = case shown="False" w578 {
              tunnel: ["Specific Argument should either be blank or\nUse Source Divertor Valve ; (wait time in seconds optional)" ""] -> w577
              frame False {
              }
              frame True {
              }
            }
          }
          frame "Check Beam Power" {
            n219 = Unbundle By Name(w588) -> ("Extra Commands"=w590:string, "Start X"=w595:dbl, "Start Y"=w593:dbl, "Start Z"=w594:dbl)
            n220 = global read "Extra_Commands_Global.vi" "Skip Traverse Position Demand"() -> (w591:string)
            n221 = call "Extra_Commands.vi"("String to Search"=w590, "Command"=w591) -> ("Command Found"=w589:bool)  [unwired: 1 in, 4 out]
            n222 = case shown="False" w589 {
              tunnel: w595 -> [w607 _]
              tunnel: w594 -> [w606 _]
              tunnel: w593 -> [w605 _]
              tunnel: "" -> [w602 w608]
              tunnel: [w601 w608] -> w587
              frame False {
                n223 = Build Array(w607, w605, w606) -> (w604:dbl[])
                n224 = Not A Number/Path/Refnum?(number/path/refnum=w604) -> (NaN/Path/Refnum?=w603:bool[])
                n225 = Or Array Elements(Boolean array=w603) -> (logical OR=w600:bool)
                n226 = Select(t="The start position is where the datum velocity measurement will be made. This should not contain NaNs.\n" ("f"), s=w600, f=w602) -> (s? t:f=w601:string)
              }
              frame True {
              }
            }
            n227 = Bundle By Name(cluster=w588, "Comments"="Start Position is the location of Datum Velocity Measurement") -> (w596:T1)
          }
          frame "Scanning Valve Measurement" {
            w622 = ext -0.5  # lo
            w623 = ext 47.5  # hi
            n228 = Unbundle By Name(w609) -> ("Specific Arguments"=w619:string)
            n229 = call "Get_array_values_fr_String.vi"("String Value"=w619) -> ("Numeric Array"=w618:dbl[], "String array"=w614:string[])
            n230 = Build Array("Averaging:Time:(mins)" ("Label for value"), "Filename:HD:Users" ("Label for value")) -> (w626:string[])
            n231 = Index Array(array=w614, index=0) -> (element=w613:string)
            n232 = Empty String/Path?(string/path=w613) -> (empty?=w611:bool)
            n233 = Index Array(array=w618, index=0) -> (element=w616:dbl)
            n234 = In Range and Coerce(upper limit=w623, x=w616, lower limit=w622) -> (In Range?=w612:bool)  [unwired: 1 out]
            n235 = Compound Arithmetic op=AND(invert w611, w612) -> (w610:bool)
            n236 = Select(t="", s=w610, f="Enter the scanning valve port number between 0 and 47 in the specific arguments box.\n") -> (s? t:f=w621:string)
          }
          frame "Set ADAM Ch" {
            n237 = Unbundle By Name(w637) -> ("Specific Arguments"=w648:string)
            n238 = while {
              shift-right: [w676] -> w644
              shift-left: _ -> [w669]
              shift-right: [w675] -> _
              shift-left: _ -> [w674]
              tunnel: w642 -> [w675]
              stop <- TRUE stop-if-true
              n239 = Array Size(array=w669) -> (size(s)=w673:i32)
              n240 = Less?(x=w675, y=w674) -> (x < y?=w671:bool)
              n241 = Equal To 0?(x=w673) -> (x = 0?=w672:bool)
              n242 = Or(x=w672, y=w671) -> (x .or. y?=w670:bool)
              n243 = case shown="True" w670 {
                tunnel: [w677 w678] -> w676
                tunnel: w669 -> [w677 _]
                frame False {
                }
                frame True {
                  n244 = call "Get_ADAM_Ch_names_client.vi"("Channel names set"=Channel_names."Active + Off") -> ("Ch names"=w678:string[])
                }
              }
            }
            n245 = call "Get_array_values_fr_String.vi"("String Value"=w648) -> ("String array"=w634:string[])  [unwired: 1 out]
            n246 = Index Array(array=w634, index=0) -> (element=w643:string)
            n247 = Search 1D Array(1D array=w644, element=w643) -> (index of element=w646:i32)  [unwired: 1 out]
            n248 = Index Array(array=w634, index=1) -> (element=w633:string)
            n249 = Empty String/Path?(string/path=w633) -> (empty?=w631:bool)
            n250 = Greater Or Equal To 0?(x=w646) -> (x >= 0?=w645:bool)
            n251 = Select(t="You have not specified a Value to Set the ADAM channel to.\nExample Specifice Argument:  ADAM_Ch_NAME  ;  10", s=w631, f="") -> (s? t:f=w629:string)
            n252 = case shown="False" w645 {
              tunnel: w644 -> [w665 _]
              tunnel: w643 -> [w663 _]
              tunnel: w642 -> [w661 _]
              tunnel: [w659 FALSE ("Cancel")] -> w641
              tunnel: w637 -> [w653 w666]
              tunnel: [w652 w666] -> w636
              tunnel: w633 -> [w650 _]
              frame False {
                n253 = Build Array(w663) -> (w662:string[])
                n254 = Format Into String(format string="Please Select the ADAM Channel that you want to set in row %d", w661) -> (resulting string=w660:string)  [unwired: 2 in, 1 out]
                n255 = call "Select_Strings.vi"("Available Ch names"=w665, "Message"=w660, "Selector mode"=T7."One", "Desired Ch names (in)"=w662) -> ("Cancel"=w659:bool, "Selected Channel Names"=w657:string[])  [unwired: 3 out]
                n256 = Index Array(array=w657, index=0) -> (element=w655:string)
                n257 = Concatenate Strings(w655, "  ;  " ("string"), w650) -> (w651:string)
                n258 = Bundle By Name(cluster=w653, "Specific Arguments"=w651) -> (w652:T1)
              }
              frame True {
              }
            }
            n259 = Select(t="Close Front Panel", s=w641, f=w639) -> (s? t:f=w640:string)
          }
          frame "Run VI Named:" {
            w691 = "Run_VI_Named_specific.vi"
            n260 = Unbundle By Name(w686) -> ("Specific Arguments"=w694:string)
            n261 = global read "Constants_global.vi" "Run VI Folder"() -> (w692:path)
            n262 = Match Pattern(string=w694, regular expression=";") -> (before substring=w695:string)  [unwired: 4 out]
            n263 = call <vilib>:"Trim Whitespace.vi"("string"=w695) -> ("trimmed string"=w687:string)  [unwired: 1 in]
            n264 = call "Run_VI_Named_specific.vi"("Run VI Named String"=w687, "Multi Run Row"=w686) -> ("Checks"=w681:string[], "Error String"=w680:string, "Check for start NaNs?"=w685:bool)  [unwired: 7 out]
            n265 = Select(t="Check for Start NaNs" ("Label for value"), s=w685, f=w683) -> (s? t:f=w682:string)
            n266 = Build Path(base path=w692, name or relative path=w687) -> (appended path=w698:path)
            n267 = Not Equal?(x=w687, y=w691) -> (x != y?=w690:bool)
            n268 = call "Does_file_exist_(simple).vi"("Pathname"=w698) -> ("exists?"=w689:bool)
            n269 = And(x=w689, y=w690) -> (x .and. y?=w688:bool)
            n270 = case shown="False" w688 {
              tunnel: [w705 ""] -> w693
              tunnel: w692 -> [w701 _]
              tunnel: w691 -> [w699 _]
              frame False {
                w703 = "\r\n"
                n271 = Build Array(w699) -> (w700:string[])
                n272 = call "List_files_in_order_of_age.vi"("Files to Hide"=w700, "Folder"=w701) -> ("file names"=w702:string[])
                n273 = for {
                  shift-right: [w709] -> w706
                  shift-left: "Cannot find the VI to run. Specific Argument options are:" -> [w710]
                  tunnel: w702 -> [w711] mode=indexing
                  w708 = "  " ("Substring")
                  n274 = Concatenate Strings(w710, w708, w711, w708) -> (w709:string)
                }
                n275 = Concatenate Strings(w706, w703, "Please place one of these strings in the \"Specific Argument\" field.", w703) -> (w705:string)
              }
              frame True {
              }
            }
            n276 = Concatenate Strings(w680, w693) -> (w697:string)
          }
          frame "Wait (minutes)" {
            n277 = Unbundle By Name(w714) -> ("Specific Arguments"=w715:string)
            n278 = call "Wait_Case_Arg.vi"("Specific Argument"=w715) -> ("Error Comments"=w716:string)  [unwired: 1 in, 4 out]
          }
          frame "Send Message" {
          }
          frame "Synchronize With:" {
            n279 = local read "Current Sync Number"() -> (w724:i32)
            n280 = call "Synchronize_Prog_Arg.vi"("Execution Row"=w723) -> ("Error Comments"=w726:string, "Sync No"=w732:i32)  [unwired: 3 out]
            n281 = Equal?(x=w732, y=w724) -> (x = y?=w731:bool)
            n282 = Format Into String(format string="This should be Synchroisation number %d.\n" ("Format String"), w724) -> (resulting string=w729:string)  [unwired: 2 in, 1 out]
            n283 = Select(t="", s=w731, f=w729) -> (s? t:f=w727:string)
            n284 = Concatenate Strings(w727, w726) -> (w725:string)
          }
          frame "Fall Back to this Row" {
          }
          frame "Turn Off Row Repeating" {
          }
          frame "Blank Row" {
            n285 = Unbundle By Name(w745) -> ("Comments"=w751:string)
            n286 = Match Pattern(string=w751, regular expression="(No Match Info)") -> (before substring=w744:string, after substring=w748:string)  [unwired: 3 out]
            n287 = Empty String/Path?(string/path=w748) -> (empty?=w749:bool)
            n288 = Bundle By Name(cluster=w745, "Comments"=w744) -> (w743:T1)
            n289 = Select(t=w748, s=w749, f="The Row Type Selector \"%s\" was not matched. Please select the desired type.\n") -> (s? t:f=w747:string)
          }
        }
        "Checks" <- w414
        n290 = Concatenate Strings(w417, w418) -> (w416:string)
      }
      frame "Sort out start and end positions" {
        n291 = Unbundle By Name(w758) -> ("Start X"=w770:dbl, "Start Y"=w769:dbl, "Start Z"=w768:dbl, "End X"=w767:dbl, "End Y"=w766:dbl, "End Z"=w765:dbl, "Extra Commands"=w754:string)
        n292 = call "Which_Trav_Setup.vi"("Extra Command String"=w754) -> ("Traverse Setup"=w753:string)
        n293 = call "Rig_Pict_Display_Pref.vi"("Traverse Name"=w753) -> ("Which Axis is vertical?"=w764:enum16{"X Axis", "Y Axis", "Z Axis"})  [unwired: 7 out]
        n294 = case shown="\"Multi-Axis Profile\", Default" w759 {
          tunnel: [w810 FALSE w826 w839 FALSE] -> w773
          tunnel: [w809 FALSE w825 w838 FALSE] -> w772
          tunnel: [w808 FALSE w824 w837 FALSE] -> w771
          tunnel: w764 -> [w807 _ w823 w836 _]
          frame "Vertical Profile" {
            n295 = case shown="\"Z Axis\"" w807 {
              tunnel: [FALSE TRUE TRUE] -> w810
              tunnel: [TRUE FALSE TRUE] -> w809
              tunnel: [TRUE TRUE FALSE] -> w808
              frame "X Axis" {
              }
              frame "Y Axis" {
              }
              frame "Z Axis" {
              }
            }
          }
          frame "Auto Calibrate" {
          }
          frame "Lateral Profile" {
            n296 = case shown="\"Y Axis\"" w823 {
              tunnel: [TRUE TRUE TRUE] -> w826
              tunnel: [TRUE TRUE FALSE] -> w825
              tunnel: [FALSE FALSE TRUE] -> w824
              frame "X Axis" {
              }
              frame "Y Axis" {
              }
              frame "Z Axis" {
              }
            }
          }
          frame "Longitudinal Profile" {
            n297 = case shown="\"Y Axis\"" w836 {
              tunnel: [FALSE FALSE FALSE] -> w839
              tunnel: [TRUE TRUE TRUE] -> w838
              tunnel: [TRUE TRUE TRUE] -> w837
              frame "X Axis" {
              }
              frame "Y Axis" {
              }
              frame "Z Axis" {
              }
            }
          }
          frame "Multi-Axis Profile", Default {
          }
        }
        n298 = Build Array(w770, w769, w768) -> (w761:dbl[])
        n299 = Build Array(w767, w766, w765) -> (w760:dbl[])
        n300 = Build Array(w773, w772, w771) -> (w762:bool[])
        "Fixed Axis" <- w762
        n301 = for {
          tunnel: w762 -> [w780] mode=indexing
          tunnel: w761 -> [w779] mode=indexing
          tunnel: w760 -> [w778] mode=indexing
          shift-right: [w775] -> w757
          shift-left: w758 -> [w776]
          i -> [w777]
          n302 = case shown="False" w780 {
            tunnel: w779 -> [_ w786]
            tunnel: w778 -> [_ w785]
            tunnel: w777 -> [_ w784]
            tunnel: w776 -> [w781 w783]
            tunnel: [w781 w782] -> w775
            frame False {
            }
            frame True {
              n303 = Not A Number/Path/Refnum?(number/path/refnum=w786) -> (NaN/Path/Refnum?=w787:bool)
              n304 = Not A Number/Path/Refnum?(number/path/refnum=w785) -> (NaN/Path/Refnum?=w789:bool)
              n305 = Exclusive Or(1:w789, 2:w787) -> (0:w788:bool)
              n306 = case shown="True" w788 {
                tunnel: w787 -> [_ w797]
                tunnel: w786 -> [_ w796]
                tunnel: w785 -> [_ w795]
                tunnel: w784 -> [_ w794]
                tunnel: w783 -> [w790 w793]
                tunnel: [w790 w792] -> w782
                frame False {
                }
                frame True {
                  n307 = Select(t=w795, s=w797, f=w796) -> (s? t:f=w791:dbl)
                  n308 = case shown="2" w794 {
                    tunnel: w793 -> [w800 w803 w806]
                    tunnel: [w799 w802 w805] -> w792
                    tunnel: w791 -> [w798 w801 w804]
                    frame 0, Default {
                      n309 = Bundle By Name(cluster=w800, "Start X"=w798, "End X"=w798) -> (w799:T1)
                    }
                    frame 1 {
                      n310 = Bundle By Name(cluster=w803, "Start Y"=w801, "End Y"=w801) -> (w802:T1)
                    }
                    frame 2 {
                      n311 = Bundle By Name(cluster=w806, "Start Z"=w804, "End Z"=w804) -> (w805:T1)
                    }
                  }
                }
              }
            }
          }
        }
      }
      frame "Check for position NaNs" {
        n312 = global read "Extra_Commands_Global.vi" "Skip Traverse Position Demand"() -> (w855:string)
        n313 = Unbundle By Name(w858) -> ("Extra Commands"=w854:string, "Start X"=w867:dbl, "Start Y"=w865:dbl, "Start Z"=w866:dbl, "End X"=w864:dbl, "End Y"=w863:dbl, "End Z"=w862:dbl)
        n314 = call "Extra_Commands.vi"("String to Search"=w854, "Command"=w855) -> ("Command Found"=w852:bool)  [unwired: 1 in, 4 out]
        n315 = case shown="False" w852 {
          tunnel: w867 -> [w882 _]
          tunnel: w866 -> [w881 _]
          tunnel: w865 -> [w880 _]
          tunnel: w864 -> [w879 _]
          tunnel: w863 -> [w878 _]
          tunnel: w862 -> [w877 _]
          tunnel: [w873 w883] -> w861
          tunnel: [w872 TRUE] -> w860
          tunnel: "" -> [w871 w883]
          frame False {
            n316 = Build Array(w882, w880, w881, w879, w878, w877) -> (w876:dbl[])
            n317 = Not A Number/Path/Refnum?(number/path/refnum=w876) -> (NaN/Path/Refnum?=w875:bool[])
            n318 = Or Array Elements(Boolean array=w875) -> (logical OR=w872:bool)
            n319 = Select(t="Some of the Start and End positions are NaN.\n" ("f"), s=w872, f=w871) -> (s? t:f=w873:string)
          }
          frame True {
          }
        }
        n320 = case shown="\"Set Tunnel Speed Only\", Default" w856 {
          tunnel: w860 -> [_ w889]
          tunnel: ["Check source details" ("t") w888] -> w859
          frame "Multi-Axis Profile" {
          }
          frame "Set Tunnel Speed Only", Default {
            n321 = Select(t="Check source details", s=w889, f="Check profile rows") -> (s? t:f=w888:string)
          }
        }
        n322 = Concatenate Strings(w869, w861) -> (w868:string)
      }
      frame "Check for Start NaNs" {
        n323 = Unbundle By Name(w895) -> ("Extra Commands"=w891:string, "Start X"=w900:dbl, "Start Y"=w898:dbl, "Start Z"=w899:dbl)
        n324 = global read "Extra_Commands_Global.vi" "Skip Traverse Position Demand"() -> (w892:string)
        n325 = call "Extra_Commands.vi"("String to Search"=w891, "Command"=w892) -> ("Command Found"=w890:bool)  [unwired: 1 in, 4 out]
        n326 = case shown="True" w890 {
          tunnel: w900 -> [w912 _]
          tunnel: w899 -> [w911 _]
          tunnel: w898 -> [w910 _]
          tunnel: "" -> [w907 w913]
          tunnel: [w905 w913] -> w896
          frame False {
            n327 = Build Array(w912, w910, w911) -> (w909:dbl[])
            n328 = Not A Number/Path/Refnum?(number/path/refnum=w909) -> (NaN/Path/Refnum?=w908:bool[])
            n329 = Or Array Elements(Boolean array=w908) -> (logical OR=w904:bool)
            n330 = Select(t="Some of the Start coordinates are NaN.\n" ("f"), s=w904, f=w907) -> (s? t:f=w905:string)
          }
          frame True {
          }
        }
        n331 = Concatenate Strings(w902, w896) -> (w901:string)
      }
      frame "Check profile rows" {
        n332 = call "Create_Pos_array.vi"("Traverse line"=w923) -> ("Traverse line Out"=w922:T1, "Error Messages"=w921:string)  [unwired: 7 out]
        n333 = Unbundle By Name(w923) -> ("Start X"=w945:dbl, "Start Y"=w944:dbl, "Start Z"=w943:dbl, "End X"=w942:dbl, "End Y"=w941:dbl, "End Z"=w940:dbl, "Specific Arguments"=w934:string, "Spacing"=w929:T2, "No. of pts."=w928:i32)
        n334 = local read "Fixed Axis"() -> (w927:bool[])
        n335 = Build Array(w945, w944, w943) -> (w925:dbl[])
        n336 = Build Array(w942, w941, w940) -> (w926:dbl[])
        n337 = case shown="\"Linear\"" w929 {
          tunnel: w934 -> [_ _ _ _ w980]
          tunnel: ["" w953 "\"N/A\" is not a valid point spacing.\n" "" w975] -> w933
          tunnel: w928 -> [_ _ _ _ w979]
          tunnel: w927 -> [_ w951 _ _ _]
          tunnel: w926 -> [_ w958 _ _ _]
          tunnel: w925 -> [_ w957 _ _ _]
          frame "Linear" {
          }
          frame "Log" {
            n338 = for {
              tunnel: w958 -> [w962] mode=indexing
              tunnel: w957 -> [w961] mode=indexing
              tunnel: [w960] -> w956 mode=indexing
              tunnel: w951 -> [w959] mode=indexing
              n339 = case shown="False" w959 {
                tunnel: w962 -> [w968 _]
                tunnel: w961 -> [w967 _]
                tunnel: [w963 FALSE] -> w960
                frame False {
                  w966 = 0.001 ("y")
                  n340 = Less?(x=w968, y=w966) -> (x < y?=w964:bool)
                  n341 = Less?(x=w967, y=w966) -> (x < y?=w965:bool)
                  n342 = Or(x=w964, y=w965) -> (x .or. y?=w963:bool)
                }
                frame True {
                }
              }
            }
            n343 = Or Array Elements(Boolean array=w956) -> (logical OR=w955:bool)
            n344 = Select(t="For log spacing, Start & End positions must be greater than 0.0001.", s=w955, f="") -> (s? t:f=w953:string)
          }
          frame "N/A" {
          }
          frame "Gauss" {
          }
          frame "Specified" {
            n345 = call "Get_array_values_fr_String.vi"("String Value"=w980) -> ("Numeric Array"=w974:dbl[])  [unwired: 1 out]
            n346 = Array Size(array=w974) -> (size(s)=w973:i32)
            n347 = Decrement(x=w973) -> (x-1=w972:i32)
            n348 = Equal?(x=w972, y=w979) -> (x = y?=w978:bool)
            n349 = Select(t="", s=w978, f="The No of points and No of Arguments do not match.\n") -> (s? t:f=w975:string)
          }
        }
        n350 = for {
          tunnel: w927 -> [w986] mode=indexing
          tunnel: w925 -> [w985] mode=indexing
          tunnel: w926 -> [w984] mode=indexing
          tunnel: [w983] -> w939 mode=indexing
          shift-right: [w981] -> w918
          shift-left: bool[] [] -> [w982]
          n351 = case shown="False" w986 {
            tunnel: w985 -> [w990 w996]
            tunnel: w984 -> [w991 w995]
            tunnel: [TRUE w994] -> w983
            tunnel: w982 -> [w988 w993]
            tunnel: [w987 w993] -> w981
            frame False {
              n352 = Not Equal?(x=w990, y=w991) -> (x != y?=w989:bool)
              n353 = Build Array (concatenate)(w988, w989) -> (w987:bool[])
            }
            frame True {
              n354 = Equal?(x=w996, y=w995) -> (x = y?=w994:bool)
            }
          }
        }
        n355 = Array Size(array=w918) -> (size(s)=w917:i32)
        n356 = And Array Elements(Boolean array=w939) -> (logical AND=w938:bool)
        n357 = Or Array Elements(Boolean array=w918) -> (logical OR=w915:bool)
        n358 = Not Equal To 0?(x=w917) -> (x != 0?=w916:bool)
        n359 = And(x=w915, y=w916) -> (x .and. y?=w914:bool)
        n360 = Select(t="", s=w938, f="This profile moves more than one axis.\n") -> (s? t:f=w935:string)
        n361 = Select(t="", s=w914, f="The start and end points are the same for this profile.\n") -> (s? t:f=w931:string)
        n362 = Concatenate Strings(w921, w931, w935, w933) -> (w948:string)
        n363 = Concatenate Strings(w947, w948) -> (w946:string)
      }
      frame "Check source details" {
        n364 = Unbundle By Name(w1008) -> ("Emission Rate (l/min)"=w1010:dbl, "Density Ratio"=w1000:string)  [unwired: 1 out]
        n365 = Empty String/Path?(string/path=w1000) -> (empty?=w1001:bool)
        n366 = Equal?(x=w1000, y="---------" ("f")) -> (x = y?=w999:bool)
        n367 = Or(x=w1001, y=w999) -> (x .or. y?=w998:bool)
        n368 = Greater Than 0?(x=w1010) -> (x > 0?=w1005:bool)
        n369 = And(x=w1005, y=w998) -> (x .and. y?=w1009:bool)
        n370 = case shown="False" w1009 {
          tunnel: w1008 -> [w1013 w1016]
          tunnel: [w1013 w1014] -> w1007
          frame False {
          }
          frame True {
            (unwired) "The Density Ratio Box should contain either:\nCarrier 1 Only\nCarrier 2 Only\nor the relative density ratio of the mixed gas with respect to air" ("f")
            n371 = Bundle By Name(cluster=w1016, "Density Ratio"="Carrier 1 Only") -> (w1014:T1)
          }
        }
        n372 = Select(t="Check source detail 2", s=w1005, f="check entered filename etc") -> (s? t:f=w1003:string)
      }
      frame "Check source detail 2" {
        n373 = Unbundle By Name(w1040) -> ("Trace Gas Concentration (%)"=w1041:dbl, "Density Ratio"=w1042:string)
        n374 = To Upper Case(1:w1042) -> (0:w1025:string)
        n375 = To Upper Case(1:"Carrier 1 Only") -> (0:w1027:string)
        n376 = To Upper Case(1:"Carrier 2 Only") -> (0:w1026:string)
        n377 = In Range and Coerce(upper limit=ext 3.01 ("hi"), x=w1041, lower limit=ext 0.0 ("lo")) -> (In Range?=w1022:bool)  [unwired: 1 out]
        n378 = Equal?(x=w1025, y=w1027) -> (x = y?=w1032:bool)
        n379 = Equal?(x=w1025, y=w1026) -> (x = y?=w1031:bool)
        n380 = Fract/Exp String To Number(string=w1025) -> (number=w1033:dbl)  [unwired: 4 out]
        n381 = In Range and Coerce(upper limit=ext 10.0 ("hi"), x=w1033, lower limit=ext 0.05 ("lo")) -> (In Range?=w1030:bool)  [unwired: 1 out]
        n382 = Compound Arithmetic op=OR(w1032, w1031, w1030) -> (w1017:bool)
        n383 = Select(t="", s=w1022, f="The Trace Gas Concentration must be within the range of 0 to 3%.\n") -> (s? t:f=w1018:string)
        n384 = Select(t="", s=w1017, f="The Density Ratio Box should contain either:\nCarrier 1 Only\nCarrier 2 Only\nor the relative density ratio of the mixed gas with respect to air") -> (s? t:f=w1019:string)
        n385 = Concatenate Strings(w1018, w1019) -> (w1043:string)
        n386 = Concatenate Strings(w1045, w1043) -> (w1044:string)
      }
      frame "check entered filename etc" {
        n387 = local read "Checks"() -> (w1058:string[])
        n388 = for {
          tunnel: w1058 -> [w1065] mode=indexing
          tunnel: [w1070] -> w1059 mode=indexing
          tunnel: w1055 -> [w1069]
          shift-right: [w1067] -> w1049
          shift-left: w1050 -> [w1068]
          tunnel: [w1066] -> w1048 mode=indexing
          n389 = case shown="\"Filename:HD:Users\"" w1065 {
            tunnel: w1068 -> [w1072 w1080 w1102 w1117]
            tunnel: [w1073 w1083 w1108 w1113] -> w1070
            tunnel: w1069 -> [_ _ w1111 _]
            tunnel: [w1072 w1080 w1100 w1117] -> w1067
            tunnel: [TRUE ("cancelled") TRUE ("cancelled") w1095 TRUE ("cancelled")] -> w1066
            tunnel: w1065 -> [_ _ _ w1115]
            frame "Number:Of:Points" {
              n390 = Unbundle By Name(w1072) -> ("No. of pts."=w1075:i32)
              n391 = Greater?(x=w1075, y=1) -> (0:w1077:bool)
              n392 = Select(t="", s=w1077, f="For a profile the number of points should be more than 1.\n" ("Format String")) -> (s? t:f=w1073:string)
            }
            frame "Averaging:Time:(mins)" {
              n393 = Unbundle By Name(w1080) -> ("Averaging time (min)"=w1082:dbl)
              n394 = Greater Than 0?(x=w1082) -> (x > 0?=w1081:bool)
              n395 = Select(t="", s=w1081, f="The averaging time should be greater than zero.\n" ("Format String")) -> (s? t:f=w1083:string)
            }
            frame "Filename:HD:Users" {
              w1109 = FALSE  # Show Error handler
              n396 = Unbundle By Name(w1102) -> ("Filename"=w1086:path, "Row No"=w1097:i32, "Row Type Selector"=w1093:T3)
              n397 = call "Row_type_selector_string.vi"("Mode"=w1093) -> ("Output string"=w1092:string)
              n398 = call "Current_Filepath.vi"("Filename in"=w1086, "Data Type"="Results") -> ("Filename Out"=w1087:path)  [unwired: 1 out]
              n399 = Path To String(path=w1087) -> (string=w1106:string)
              n400 = Not A Number/Path/Refnum?(number/path/refnum=w1087) -> (NaN/Path/Refnum?=w1090:bool)
              n401 = Equal?(x=Multi_run_mode."Run VI Named:" ("Mode"), y=w1111) -> (x = y?=w1110:bool)
              n402 = Match Pattern(string=w1106, regular expression="-------" ("f")) -> (match substring=w1105:string)  [unwired: 4 out]
              n403 = Empty String/Path?(string/path=w1105) -> (empty?=w1091:bool)
              n404 = Format Into String(format string=" For Row  %d %s." ("Comment"), w1097, w1092) -> (resulting string=w1096:string)  [unwired: 2 in, 1 out]
              n405 = Compound Arithmetic op=AND(w1091, invert w1090) -> (w1089:bool)
              n406 = Select(t=w1087, s=w1089, f=path "") -> (s? t:f=w1104:path)
              n407 = call "Results_filename_checker.vi"("Filelength"=45, "Warn if Already Exists"=w1110, "Comment"=w1096, "Show Error handler"=w1109, "Results file"=w1104) -> ("Error String"=w1108:string, "cancelled"=w1099:bool, "Results file output"=w1101:path)  [unwired: 1 out]
              n408 = Bundle By Name(cluster=w1102, "Filename"=w1101) -> (w1100:T1)
              n409 = Not(x=w1099) -> (.not. x?=w1095:bool)
            }
            frame "No Match", Default {
              n410 = Concatenate Strings(w1115, " Has not been programmed.\n" ("string")) -> (w1113:string)
            }
          }
        }
        n411 = local read "Editted Row"() -> (w1052:bool)
        n412 = And Array Elements(Boolean array=w1048) -> (logical AND=w1047:bool)
        n413 = Concatenate Strings(w1059) -> (w1057:string)
        n414 = Concatenate Strings(w1056, w1057) -> (w1051:string)
        n415 = Empty String/Path?(string/path=w1051) -> (empty?=w1054:bool)
        n416 = case shown="False" w1054 {
          tunnel: ["Open Front Panel" w1063] -> w1053
          tunnel: w1052 -> [_ w1064]
          frame False {
          }
          frame True {
            n417 = Select(t="Close Front Panel", s=w1064, f="End") -> (s? t:f=w1063:string)
          }
        }
      }
      frame "Open Front Panel" {
        w1122 = TRUE  # Front Panel Window:Open
        n418 = Current VI's Path() -> (path=w1123:path)
        n419 = call "Open_Close_Front_Panel.ph.vi"("Front Panel Window:Open"=w1122, "VI path"=w1123) -> ()  [unwired: 2 out]
        n420 = local write "Editted Row"(TRUE ("Editted Row")) -> ()
        n421 = local write "Execution Row"(w1119) -> ()
      }
      frame "What to do next?" {
        w1133 = ""
        w1131 = "[\r\n]"
        n422 = local read "Execution Row"() -> (w1129:T1)
        n423 = Unbundle By Name(w1129) -> ("Row Type Selector"=w1145:T3, "Specific Arguments"=w1140:string, "Extra Commands"=w1138:string, "Density Ratio"=w1132:string)
        n424 = Wait Until Next ms Multiple(millisecond multiple=u32 100) -> ()  [unwired: 1 out]
        n425 = Not Equal?(x=Multi_run_mode."Blank Row" ("Mode"), y=w1145) -> (x != y?=w1141:bool)
        n426 = call "Replace_Character.vi"("Replace with"=w1133, "Input String"=w1140, "Search For"=w1131) -> ("Output string"=w1139:string)  [unwired: 1 out]
        n427 = call "Replace_Character.vi"("Replace with"=w1133, "Input String"=w1138, "Search For"=w1131) -> ("Output string"=w1137:string)  [unwired: 1 out]
        n428 = call "Replace_Character.vi"("Replace with"=w1133, "Input String"=w1132, "Search For"=w1131) -> ("Output string"=w1130:string)  [unwired: 1 out]
        n429 = Compound Arithmetic op=OR("Edit in Excel", "OK") -> (w1142:bool)
        n430 = Bundle By Name(cluster=w1129, "Specific Arguments"=w1139, "Extra Commands"=w1137, "Density Ratio"=w1130) -> (w1127:T1)
        n431 = Compound Arithmetic op=AND(w1142, w1141) -> (w1135:bool)
        n432 = Not Equal?(x=w1127, y=w1129) -> (x != y?=w1128:bool)
        n433 = Not(x="Edit in Excel") -> (.not. x?=w1126:bool)
        n434 = case shown="True" w1128 {
          tunnel: w1127 -> [_ w1149]
          frame False {
          }
          frame True {
            n435 = local write "Execution Row"(w1149) -> ()
          }
        }
        n436 = case shown="True" w1126 {
          tunnel: ["Close Front Panel" w1154] -> w1134
          tunnel: w1135 -> [_ w1153]
          frame False {
          }
          frame True {
            n437 = Select(t="Clean Up Row", s=w1153, f="What to do next?") -> (s? t:f=w1154:string)
          }
        }
        "Error Comments" <- w1136
      }
      frame "Clean Up Row" {
        n438 = call "Traverse_Control_Ch_Names.vi"("Mode"=T4."All Channel Names") -> ("Channel names"=w1163:string[])  [unwired: 1 in]
        n439 = call "Trav_Cluster_to_Row.vi"("Traverse line in"=w1158, "Row Number"=w1159, "Channel names"=w1163) -> ("Traverse line Out"=w1161:T1)  [unwired: 4 out]
      }
      frame "Close Front Panel" {
        w1167 = FALSE  # Front Panel Window:Open
        n440 = Current VI's Path() -> (path=w1168:path)
        n441 = call "Open_Close_Front_Panel.ph.vi"("Front Panel Window:Open"=w1167, "VI path"=w1168) -> ()  [unwired: 2 out]
      }
      frame "End" {
        n442 = local read "Editted Row"() -> (w1176:bool)
        n443 = case shown="True" w1176 {
          tunnel: w1175 -> [w1179 w1182]
          tunnel: [w1179 w1181] -> w1173
          tunnel: w1174 -> [_ w1180]
          frame False {
          }
          frame True {
            n444 = call "Traverse_Control_Ch_Names.vi"("Mode"=T4."All Channel Names") -> ("Channel names"=w1183:string[])  [unwired: 1 in]
            n445 = call "Trav_Cluster_to_Row.vi"("Traverse line in"=w1182, "Row Number"=w1180, "Channel names"=w1183) -> ("Traverse line Out"=w1181:T1)  [unwired: 4 out]
          }
        }
        n446 = local write "Error Comments"(w1177) -> ()
      }
    }
    "Traverse line Out" <- w8
  }
  "Execution Row Out" <- w2
  "Continue?" <- w1
